vi "Kinesis - KDC101 - Move Absolute.vi"() -> ()   [LabVIEW 2012]
doc: "Shows how to move a motor to an absolute position."
uses:
  U:/Kinesis LabVIEW Website Examples/Thorlabs.MotionControl.Controls.dll
  Thorlabs.MotionControl.Controls.dll
  U:/Kinesis LabVIEW Website Examples/ThorLabs.MotionControl.KCube.DCServoCLI.dll
  ThorLabs.MotionControl.KCube.DCServoCLI.dll
panel:
  in  "SerialNumber":string
  in  "Abs Pos":dbl
  in  "Home":bool
  in  "MoveAbsolute":bool
  in  "Set Abs Pos":bool
  in  "?":bool
  in  "KCubeDCServoControl":refnum<k24>(container)
  # "Notes:"
  # "- Ensure that the appropriate .DLLs are copied into your Project Folder. Check that the correct bit type are used depending on your version of LabVIEW\ni.e. 32-bit or 64-bit.\n\n\n\n\n\n\n\n\n\n\n\n\n\n\n- Open the example VI through the LabVIEW Project Explorer to correctly load the User Interface from Thorlabs.MotionControl.Controls.dll."
  # "Thorlabs Hardware: KDC101 - K-Cube Brushless DC Servo Motor Controller\nhttps://www.thorlabs.com/thorproduct.cfm?partnumber=KDC101\n\nDescription: This VI will enable you to communicate with KDC101 to control DC Brushed Stages & Actuators. The VI will allow you to home the   device, and move it to any position without having to use the UI.\n\nInstructions: \n1) Connect your KDC101 device to your PC & power the device, ensuring your stage/actutator is connected. For full device setup, the device product manual can be found on our website here. - https://www.thorlabs.com/thorproduct.cfm?partnumber=KDC101\n2) Enter the device serial number below.\n3) Click 'Run' in the LabVIEW Toolbar.\n4) To end the Program click 'STOP'"
  # "Example Image of .NET Controller - VI opened via Project Explorer/ not opened via Project Explorer"
  # "VI Not Opened via Project Explorer"
  # "VI Opened via Project Explorer"
  # "- To explore the range of methods available, please visit the .NET API, included with your Kinesis software.\n\n- For tips on building your own VIs with Thorlabs Motion Control Hardware, please see our LabVIEW Guide here.\nhttps://www.thorlabs.com/newgrouppage9.cfm?objectgroup_id=10285"
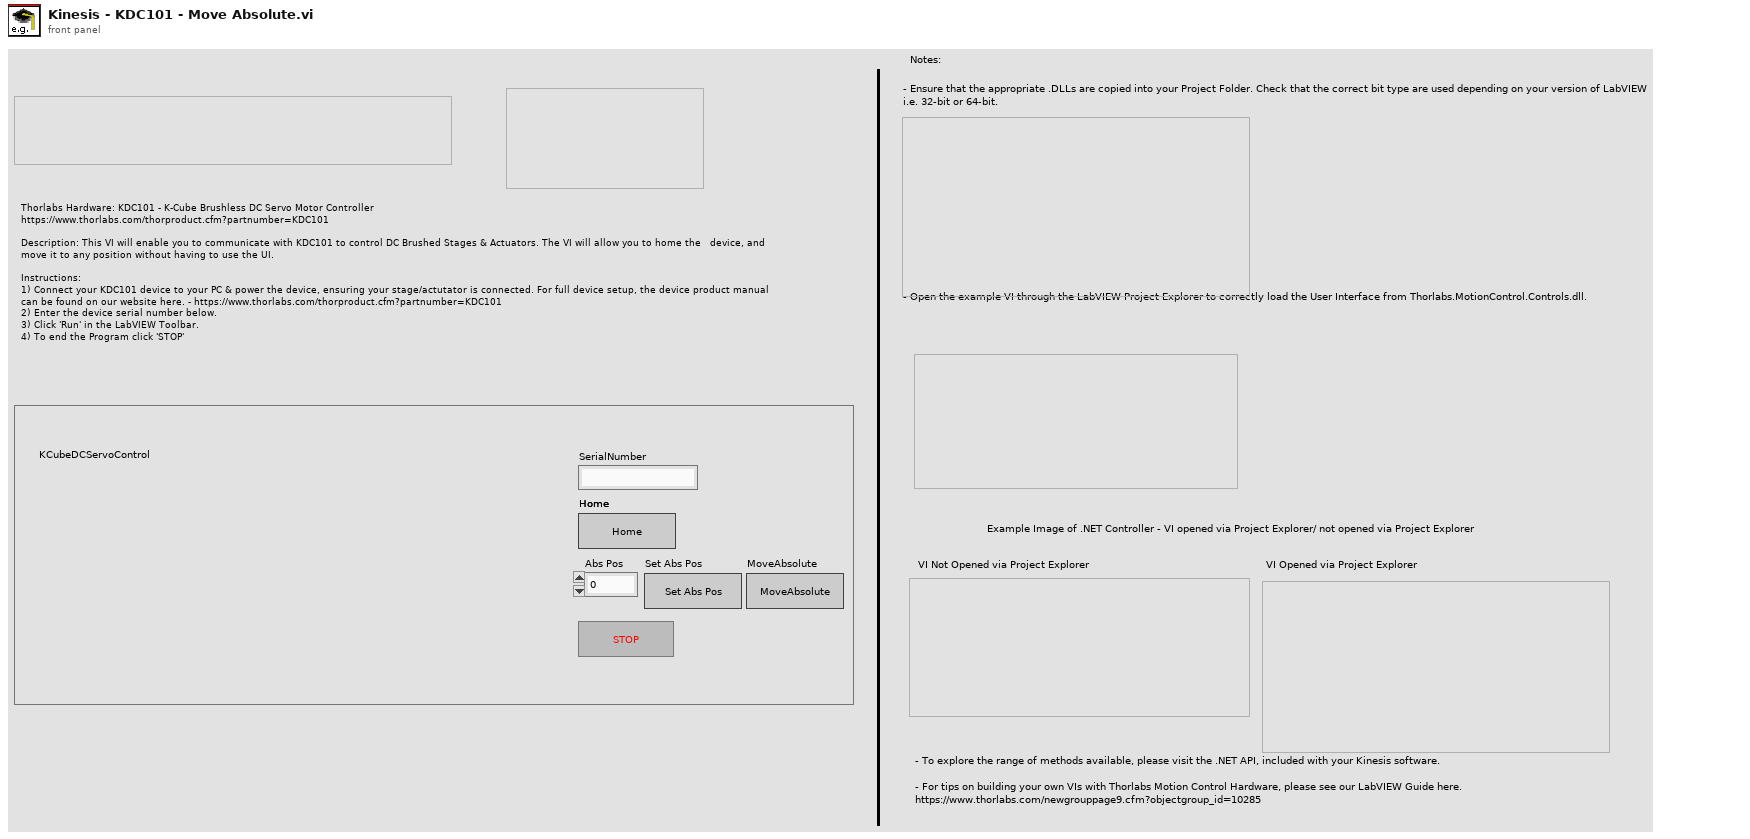
[diagram p1: front panel]
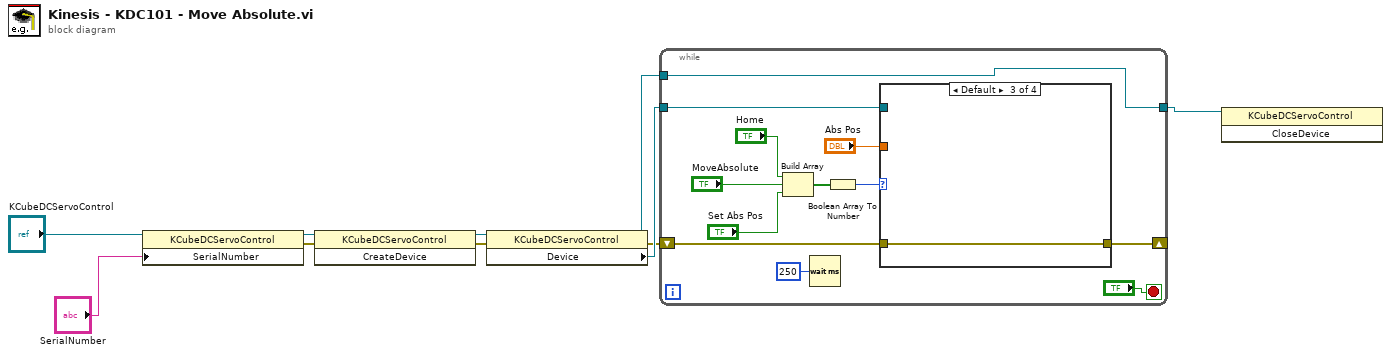
[diagram p0: block diagram]
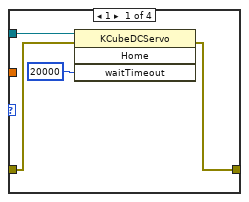
[diagram p2: hidden frame]
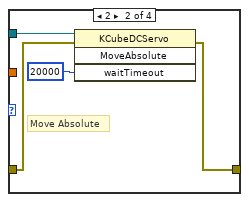
[diagram p3: hidden frame]
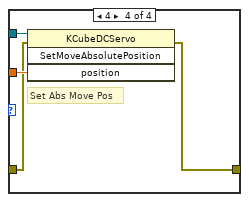
[diagram p4: hidden frame]
diagram:
  n1 = property class="KCubeDCServoControl"(reference="KCubeDCServoControl", "SerialNumber"="SerialNumber") -> (reference out=w9:refnum<k24>, error out=w6:errorcluster)  [unwired: 1 in]
  n2 = invoke class="KCubeDCServoControl" method="CreateDevice"(reference=w9, error in=w6) -> (reference out=w8:refnum<k24>, error out=w5:errorcluster)  [unwired: 1 in, 1 out]
  n3 = property class="KCubeDCServoControl"(reference=w8, error in=w5) -> (reference out=w2:refnum<k24>, error out=w4:errorcluster, "Device"=w7:refnum<k24>)
  n4 = while {
    tunnel: [w12] -> w1
    tunnel: w7 -> [w18]
    shift-right: [w15] -> _
    shift-left: w4 -> [w14]
    tunnel: w2 -> [w12]
    stop <- "?" stop-if-true
    n5 = Build Array("Home", "MoveAbsolute", "Set Abs Pos") -> (w17:bool[])
    n6 = Wait (ms)(milliseconds to wait=u32 250) -> ()  [unwired: 1 out]
    n7 = Boolean Array To Number(Boolean array=w17) -> (number=w16:u32)
    n8 = case shown="Default" w16 {
      tunnel: w18 -> [w26 w29 _ w35]
      tunnel: [w23 w27 w31 w32] -> w15
      tunnel: w14 -> [w24 w28 w31 w33]
      tunnel: "Abs Pos" -> [_ _ _ w34]
      frame 1 {
        n9 = invoke class="KCubeDCServo" method="Home"(reference=w26, error in=w24, "waitTimeout"=20000) -> (error out=w23:errorcluster)  [unwired: 1 in, 3 out]
      }
      frame 2 {
        # "Move Absolute"
        n10 = invoke class="KCubeDCServo" method="MoveAbsolute"(reference=w29, error in=w28, "waitTimeout"=20000) -> (error out=w27:errorcluster)  [unwired: 1 in, 3 out]
      }
      frame Default {
      }
      frame 4 {
        # "Set Abs Move Pos"
        n11 = invoke class="KCubeDCServo" method="SetMoveAbsolutePosition"(reference=w35, error in=w33, "position"=w34) -> (error out=w32:errorcluster)  [unwired: 1 in, 3 out]
      }
    }
  }
  n12 = invoke class="KCubeDCServoControl" method="CloseDevice"(reference=w1) -> ()  [unwired: 2 in, 3 out]
